vi "SMS Candidate Selection - Locations to ROIs.vi"(0 "Image Ref":T2, 7 "Row Column Indices":i32[][](array[numeric]), 11 "Error":errorcluster, 13 "Box Half Size":u8) -> (4 "Image Ref (DUP)":T2, 6 "Image ROIs":T1, 8 "ROI Coordinates (Left, Top, Right, Bottom)":i32[][](array[numeric]), 15 "Error Out":errorcluster)   [LabVIEW 2016]
uses:
  <vilib>/vision/Image Controls.llb/IMAQ Image.ctl
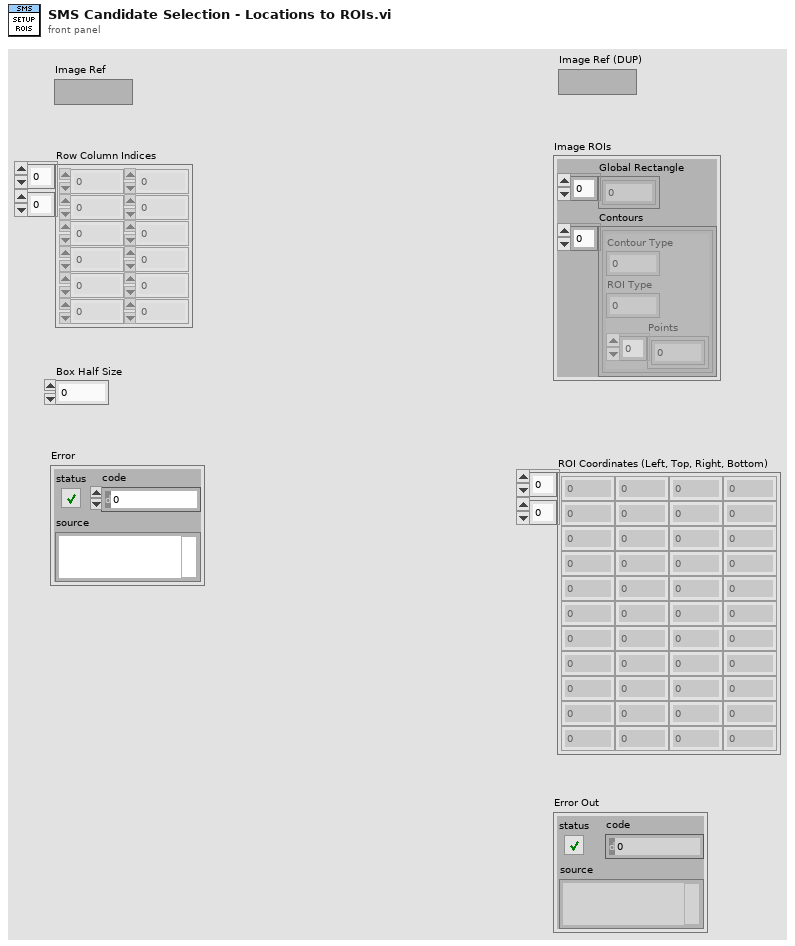
[diagram p1: front panel]
types:
  T1 = cluster{"Global Rectangle":i32[], "Contours":cluster{"Contour Type":u32, "ROI Type":u32, "Points":i32[]}[]}
  T2 = typedef "IMAQ Image.ctl" = refnum<image>
  T3 = cluster{"Contour Type":u32, "ROI Type":u32, "Points":i32[]}
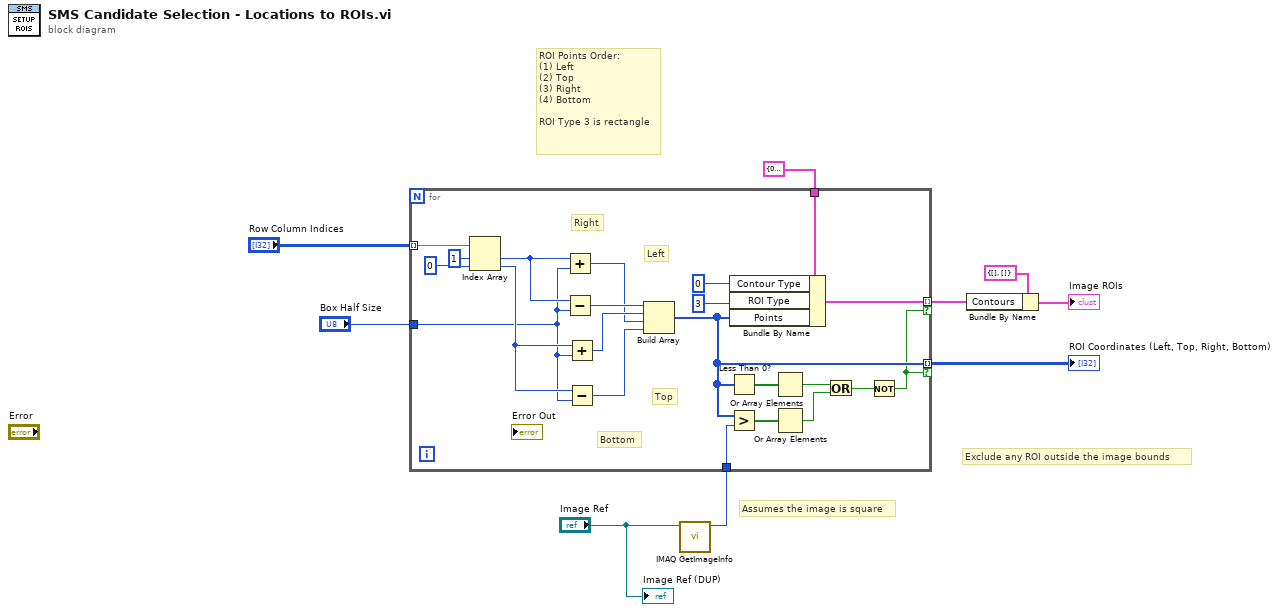
[diagram p0: block diagram]
diagram:
  # "Exclude any ROI outside the image bounds"
  # "Assumes the image is square"
  # "ROI Points Order:\n(1) Left\n(2) Top\n(3) Right\n(4) Bottom\n\nROI Type 3 is rectangle"
  n1 = call "IMAQ GetImageInfo"("Image"="Image Ref") -> ("X Resolution"=w5:i32)  [unwired: 3 in, 7 out]
  n2 = for {
    tunnel: "Row Column Indices" -> [w31] mode=indexing
    tunnel: "Box Half Size" -> [w26]
    tunnel: T3 {"Contour Type"=0, "ROI Type"=0, "Points"=[]} -> [w21]
    tunnel: [w18] -> w6 mode=indexing if=w10
    tunnel: w5 -> [w17]
    tunnel: [w11] -> w4 mode=indexing if=w10
    # "Bottom"
    # "Top"
    # "Left"
    # "Right"
    n3 = Index Array(array=w31, index #1=1 ("index"), index #2=0 ("index")) -> (element #1=w28:i32, element #2=w27:i32)
    n4 = Add(x=w28, y=w26) -> (x+y=w23:i32)
    n5 = Subtract(x=w28, y=w26) -> (x-y=w25:i32)
    n6 = Add(x=w27, y=w26) -> (x+y=w24:i32)
    n7 = Subtract(x=w27, y=w26) -> (x-y=w22:i32)
    n8 = Build Array(w25, w24, w23, w22) -> (w11:i32[])
    n9 = Less Than 0?(x=w11) -> (x < 0?=w16:bool[])
    n10 = Greater?(x=w11, y=w17) -> (0:w15:bool[])
    n11 = Bundle By Name(cluster=w21, "Contour Type"=u32 0, "ROI Type"=u32 3, "Points"=w11) -> (w18:T3)
    n12 = Or Array Elements(Boolean array=w16) -> (logical OR=w14:bool)
    n13 = Or Array Elements(Boolean array=w15) -> (logical OR=w13:bool)
    n14 = Or(x=w14, y=w13) -> (x .or. y?=w12:bool)
    n15 = Not(x=w12) -> (.not. x?=w10:bool)
  }
  "ROI Coordinates (Left, Top, Right, Bottom)" <- w4
  n16 = Bundle By Name(cluster=T1 {"Global Rectangle"=[], "Contours"=[]} ("ROI"), "Contours"=w6) -> (→"Image ROIs":T1)
  "Image Ref (DUP)" <- "Image Ref"
